vi "connect to endpoint.vi"(8 "error in":errorcluster, 10 "address":string, 11 "socket":i64) -> (0 "error out":errorcluster, 3 "endpoint":i32)   [LabVIEW 2013, in "lvnano.lvlib"]
doc: "NN_EXPORT int nn_connect (int s, const char *addr);"
uses:
  lvnano.lvlib
  lvnanomsg.dll
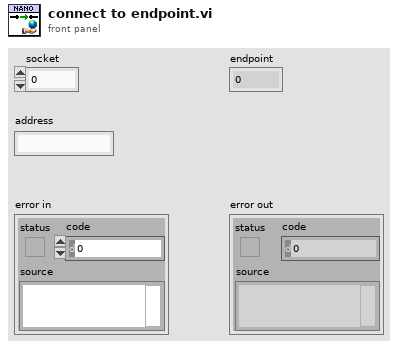
[diagram p1: front panel]
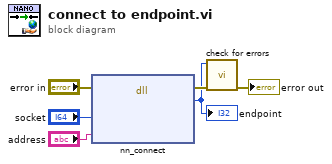
[diagram p0: block diagram]
diagram:
  n1 = dll-call lib="C:/Users/Daniel/Documents/nanomsg/lvnano/lvnanomsg.*" fn="nn_connect"(error in="error in", "socket"="socket", "address"="address") -> (error out=w3:errorcluster, "endpoint"=w1:i32)  [unwired: 4 in, 1 out]
  "endpoint" <- w1
  n2 = call "check for errors.vi"("error in"=w3, "function return"=w1) -> ("error out"=→"error out":errorcluster)  [unwired: 9 in]
